vi "SetRandomPoint.vi"(8 "error in (no error)":errorcluster, 11 "Snake in":refnum<class "Snake.lvclass">) -> (0 "error out":errorcluster, 3 "Snake out":refnum<class "Snake.lvclass">)   [LabVIEW 2019, in "RT_Game.lvlib" / "Snake.lvclass"]
uses:
  Snake.lvclass
  Snake.lvclass/Snake.ctl
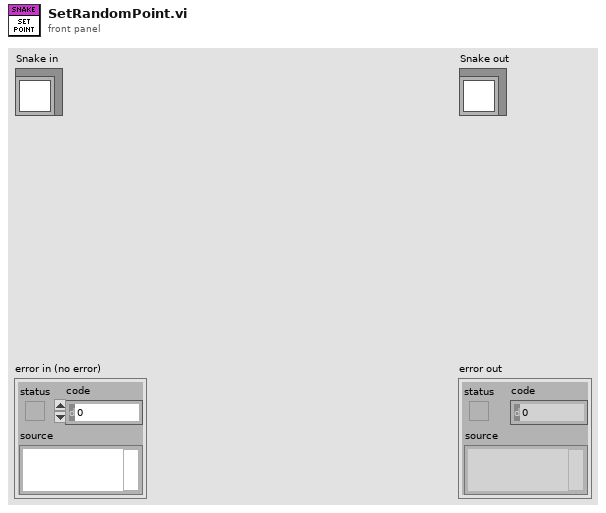
[diagram p1: front panel]
types:
  T1 = typedef "RT_Game.lvlib/Snake.lvclass/CoordinateData.ctl" = cluster{"Coordinate":T2, "TileCodes":T3}
  T2 = typedef "RT_Game.lvlib/Game.lvclass/Coordinate.ctl" = cluster{"x":i16, "y":i16}
  T3 = typedef "RT_Game.lvlib/Game.lvclass/TileCodes.ctl" = enum16{"line_vert", "line_hor", "line_rightup", "line_rightdown", "line_leftup", "line_leftdown", "bg1", "bg2", "bg3", "bg4", "bg5", "bg6", "bg7"}
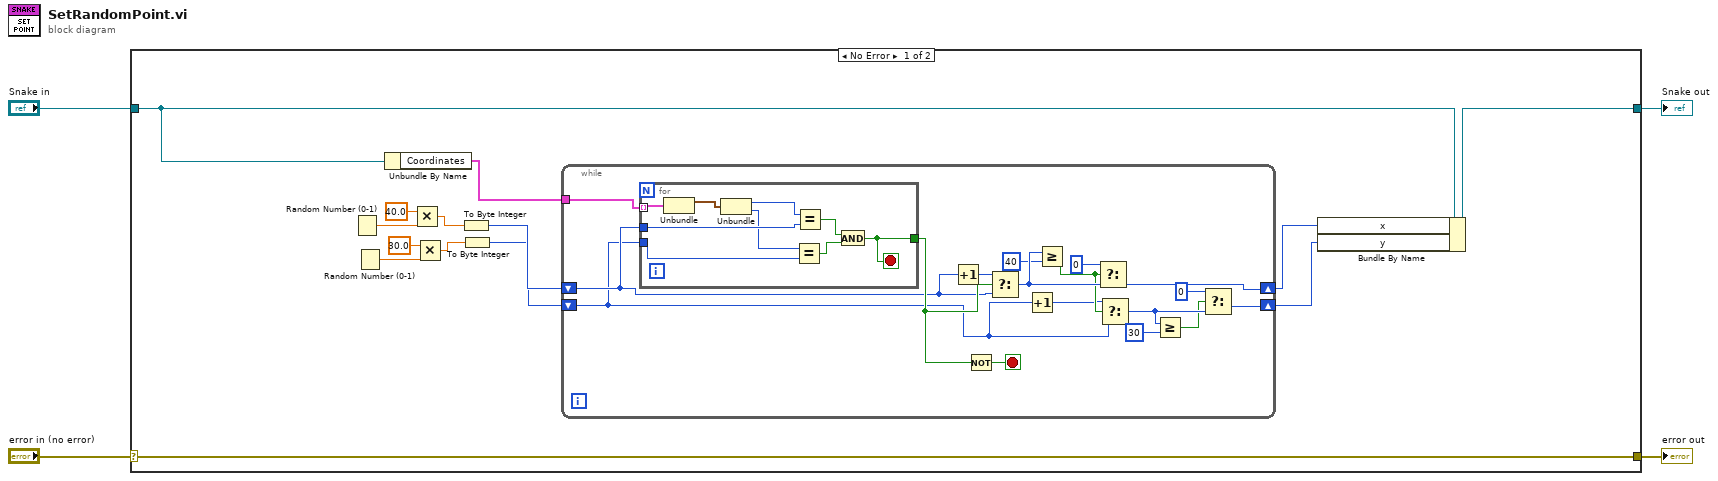
[diagram p0: block diagram]
diagram:
  n1 = case shown="No Error" "error in (no error)" {
    selector: "error in (no error)" -> [w18 w46]
    tunnel: [w18 w46] -> w3
    tunnel: [w17 w45] -> w1
    tunnel: "Snake in" -> [w10 w45]
    frame No Error {
      n2 = Random Number (0-1)() -> (number: 0 to 1=w16:dbl)
      n3 = Random Number (0-1)() -> (number: 0 to 1=w12:dbl)
      n4 = Unbundle By Name(w10) -> ("Coordinates"=w7:T1[])
      n5 = Multiply(x=40.0, y=w16) -> (x*y=w14:dbl)
      n6 = Multiply(x=30.0, y=w12) -> (x*y=w11:dbl)
      n7 = To Byte Integer(number=w14) -> (8bit integer=w9:i8)
      n8 = To Byte Integer(number=w11) -> (8bit integer=w8:i8)
      n9 = while {
        shift-right: [w28] -> w6
        shift-left: w9 -> [w32]
        shift-right: [w21] -> w5
        shift-left: w8 -> [w25]
        tunnel: w7 -> [w35]
        stop <- w33 stop-if-true
        n10 = for {
          tunnel: w35 -> [w44] mode=indexing
          tunnel: w32 -> [w43]
          tunnel: w25 -> [w42]
          tunnel: [w39] -> w34
          stop <- w39 stop-if-true
          n11 = Unbundle(w44) -> ("Coordinate"=w38:T2)  [unwired: 1 out]
          n12 = Unbundle(w38) -> ("x"=w37:i16, "y"=w36:i16)
          n13 = Equal?(x=w36, y=w42) -> (x = y?=w41:bool)
          n14 = Equal?(x=w37, y=w43) -> (x = y?=w40:bool)
          n15 = And(x=w40, y=w41) -> (x .and. y?=w39:bool)
        }
        n16 = Increment(x=w32) -> (x+1=w31:i8)
        n17 = Not(x=w34) -> (.not. x?=w33:bool)
        n18 = Select(t=w31, s=w34, f=w32) -> (s? t:f=w30:i8)
        n19 = Increment(x=w25) -> (x+1=w24:i8)
        n20 = Greater Or Equal?(x=w30, y=i8 40 ("x")) -> (x >= y?=w26:bool)
        n21 = Select(t=i8 0, s=w26, f=w30) -> (s? t:f=w28:i8)
        n22 = Select(t=w24, s=w26, f=w25) -> (s? t:f=w23:i8)
        n23 = Greater Or Equal?(x=w23, y=i8 30) -> (x >= y?=w20:bool)
        n24 = Select(t=i8 0, s=w20, f=w23) -> (s? t:f=w21:i8)
      }
      n25 = Bundle By Name(cluster=w10, "x"=w6, "y"=w5) -> (w17:refnum<class "Snake.lvclass">)
    }
    frame Error {
    }
  }
  "error out" <- w3
  "Snake out" <- w1
